vi "Patent.vi"() -> ()   [LabVIEW 2014]
uses:
  <vilib>/Instr/_visa.llb/VISA Configure Serial Port (Instr).vi
panel:
  out "flash":bool=TRUE
  out "RLCValue*":dbl=0.01
  out "Offset":string="0,00V"
  out "F4":bool
  out "F3":bool=TRUE
  out "F2":bool
  out "F1":bool
  out "Frequency":string="1kHz"
  out "Level":string="1,00V"
  out "DQValue":string="-0,0633   "
  out "RLCValue":string="0,01 pF"
  in  "Menu":bool
  in  "Down":bool
  in  ">0<":bool
  in  "F4":bool
  in  "Right":bool
  in  "Enter":bool
  in  "Left":bool
  in  "F3":bool
  in  "Z/T":bool
  in  "Up":bool
  in  "I":bool
  in  "F2":bool
  in  "R/D":bool
  in  "L/Q":bool
  in  "C/D":bool
  in  "F1":bool
  out "Ошибка связи":bool
  out "DQ":string="D"
  out "Корректный  пакет":bool=TRUE
  in  "Stop":bool
  out "Level":dbl=1.0
  out "Limit":string="A 10MOm"
  out "RLC":string="Cp"
  # "Измеритель иммитанса Е7-20"
  # "МНИПИ"
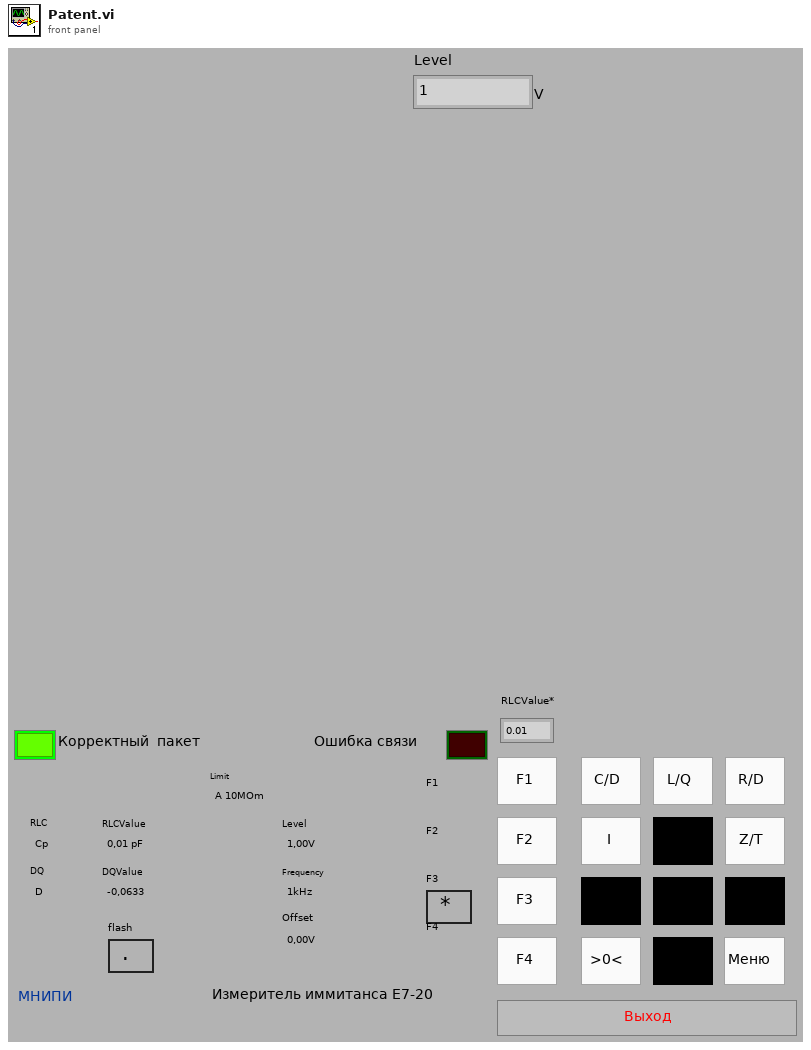
[diagram p1: front panel]
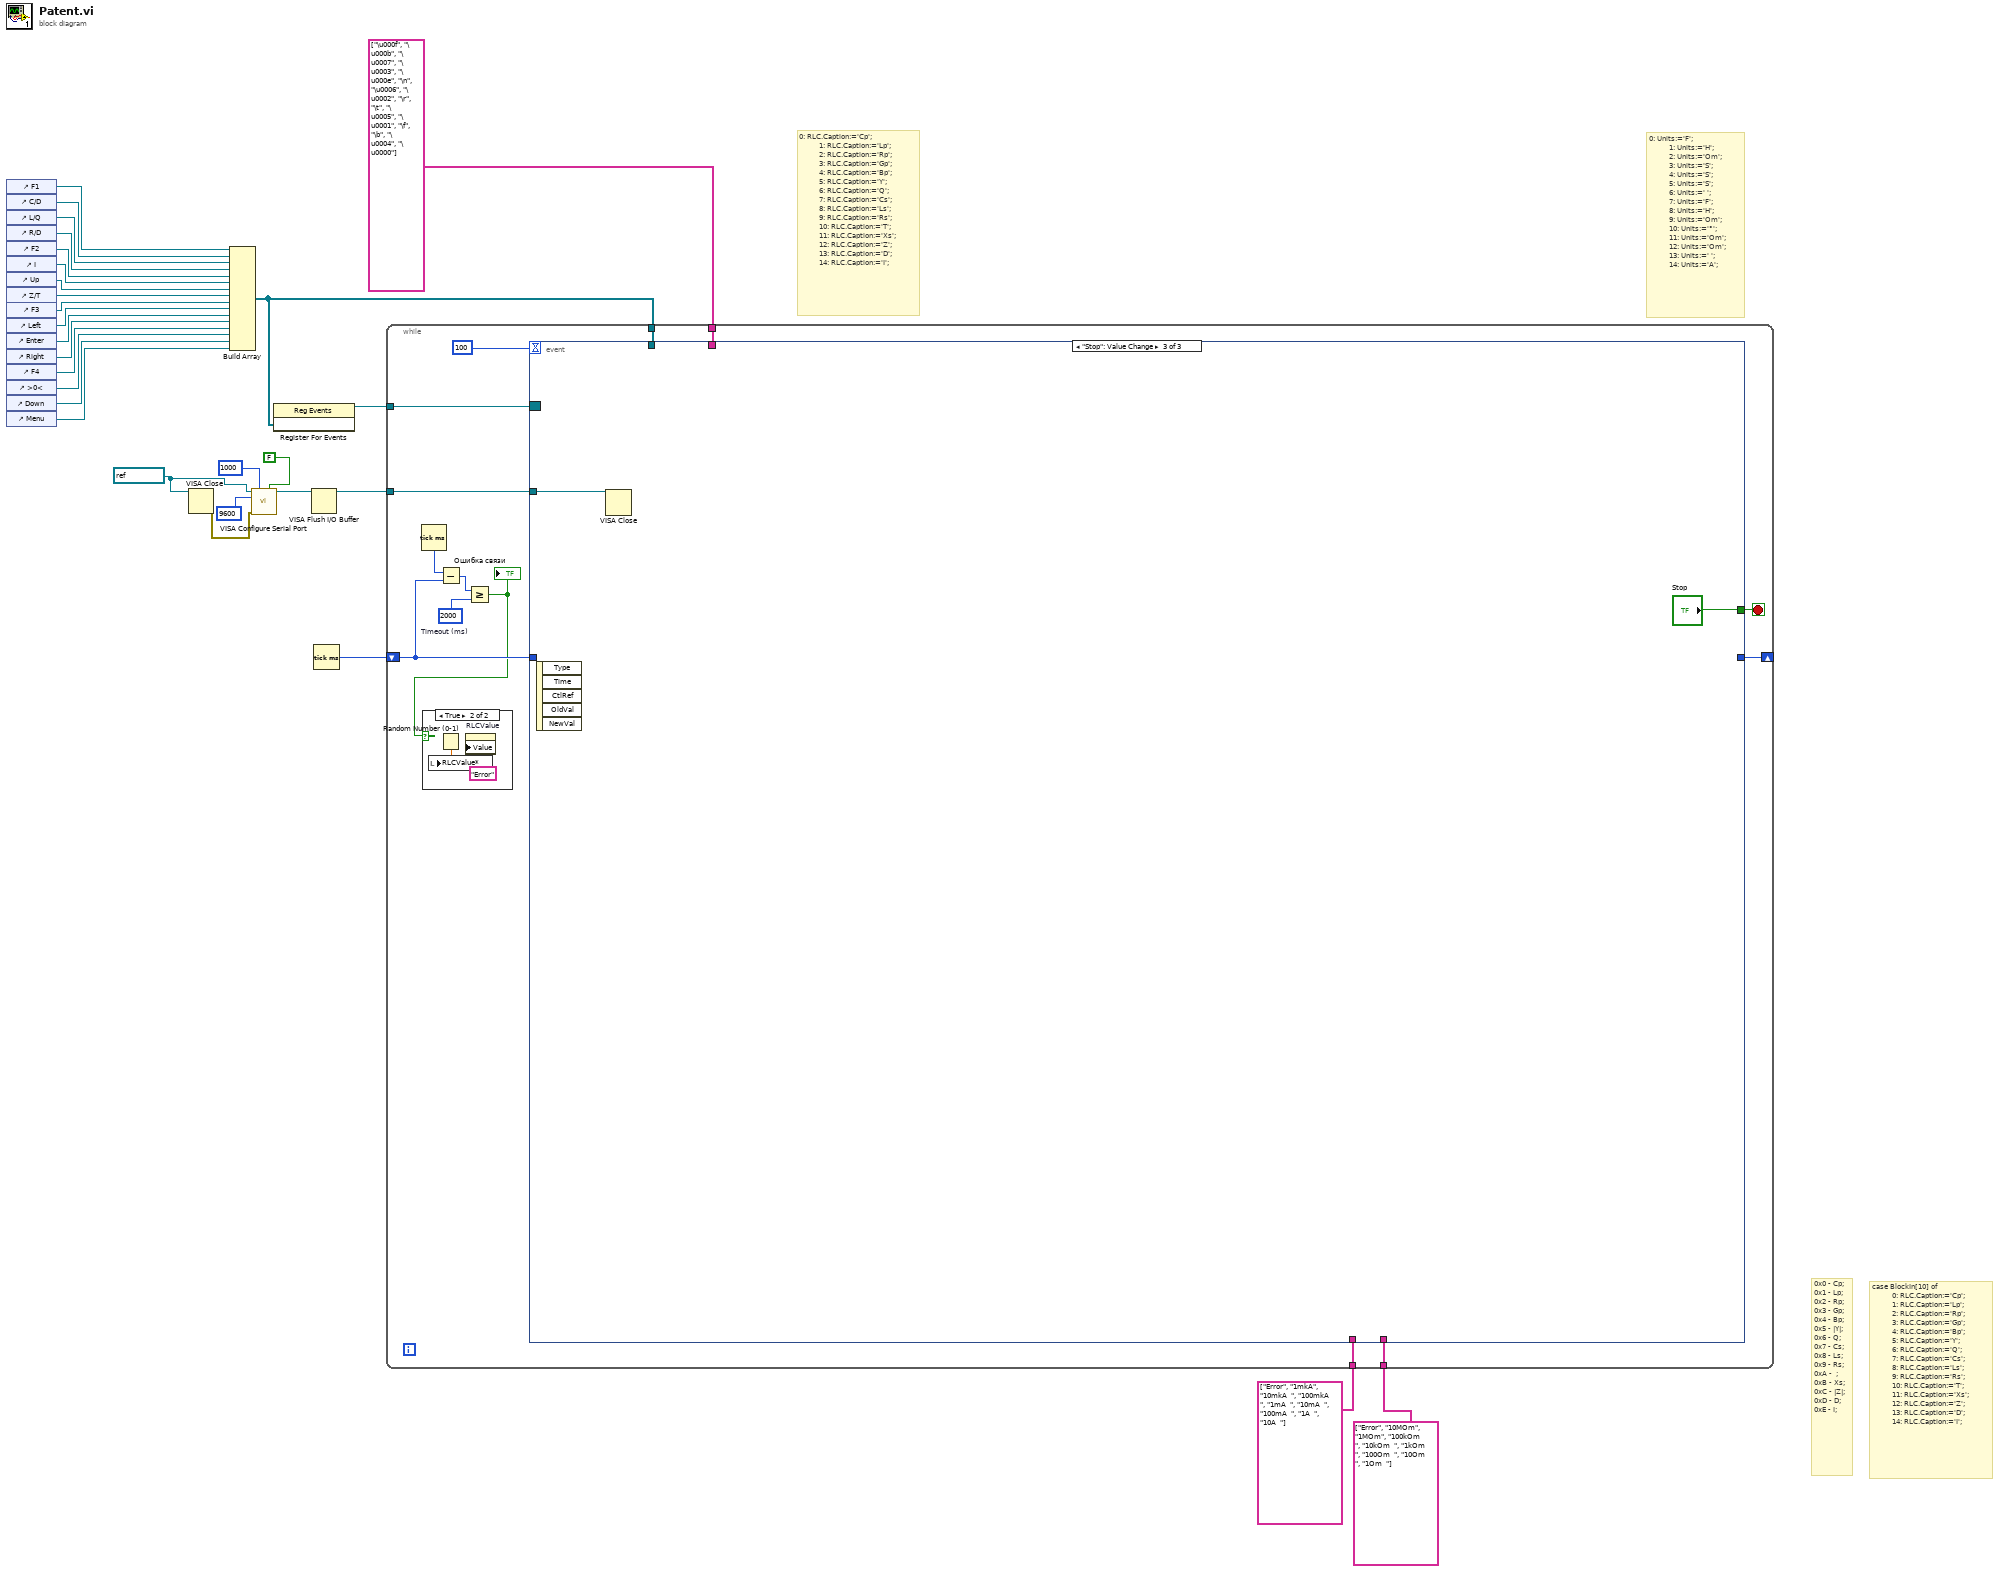
[diagram p0: block diagram]
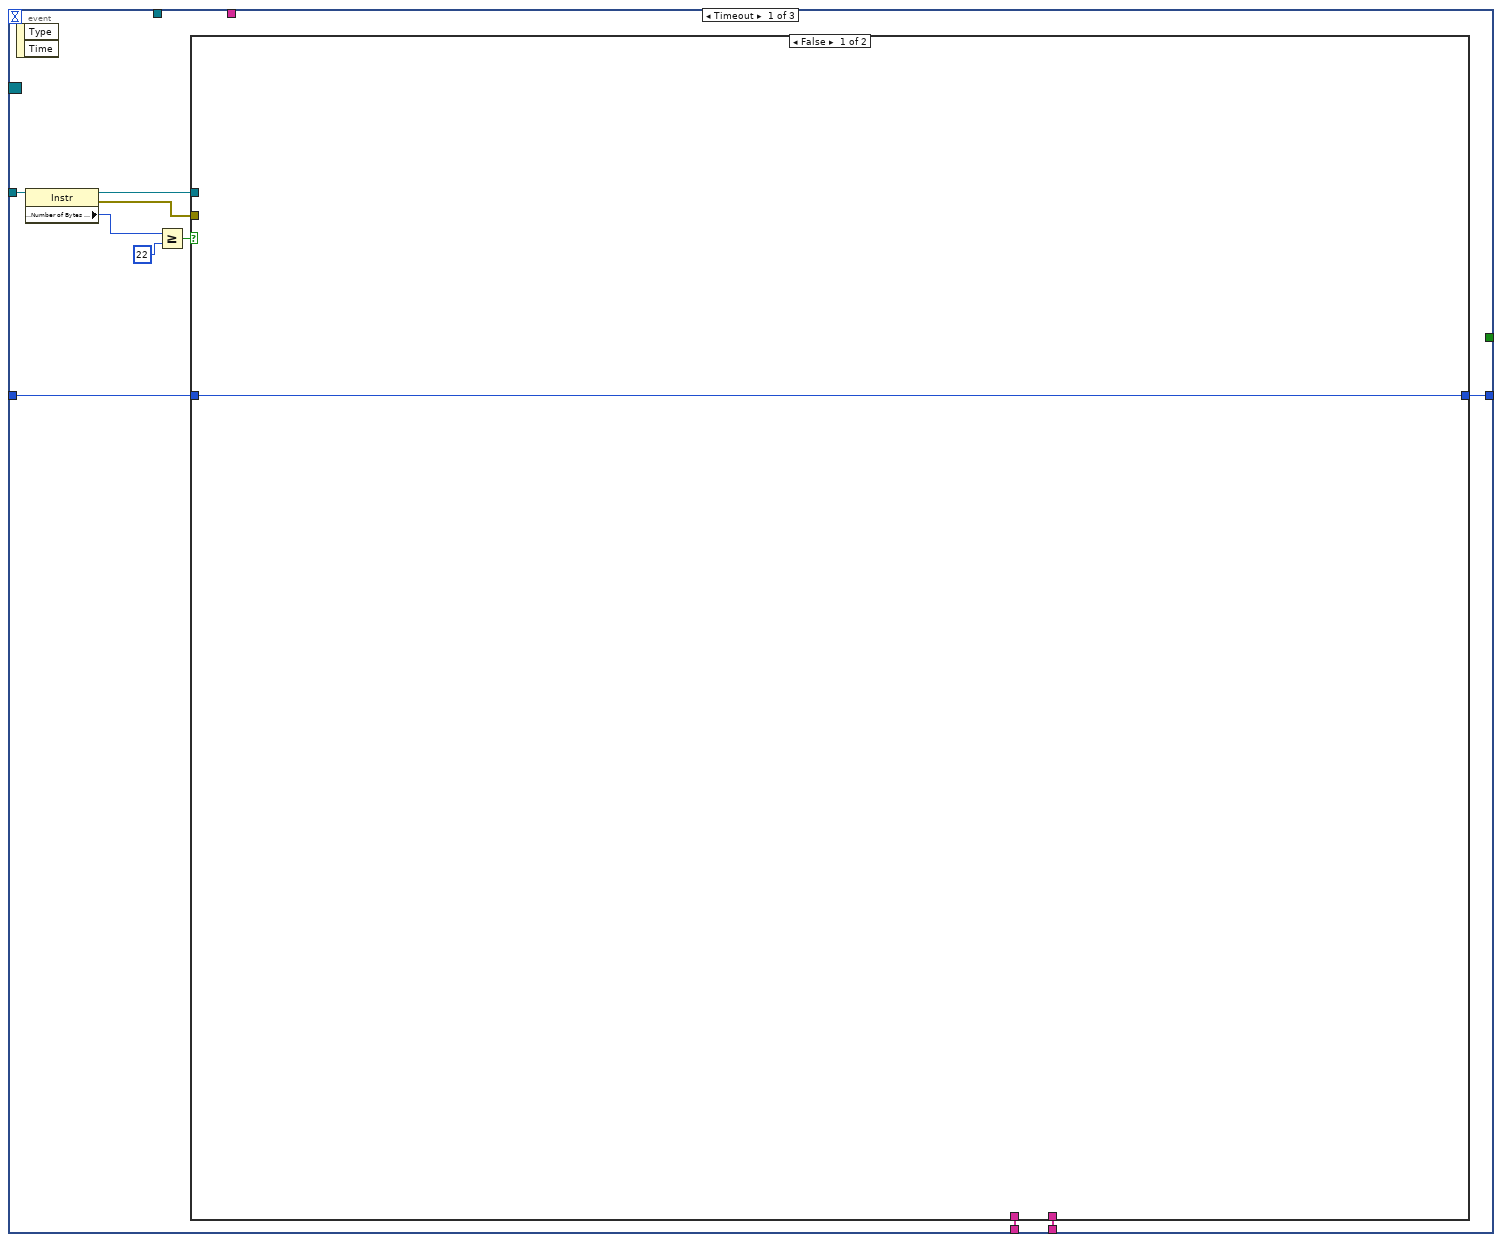
[diagram p3: hidden frame]
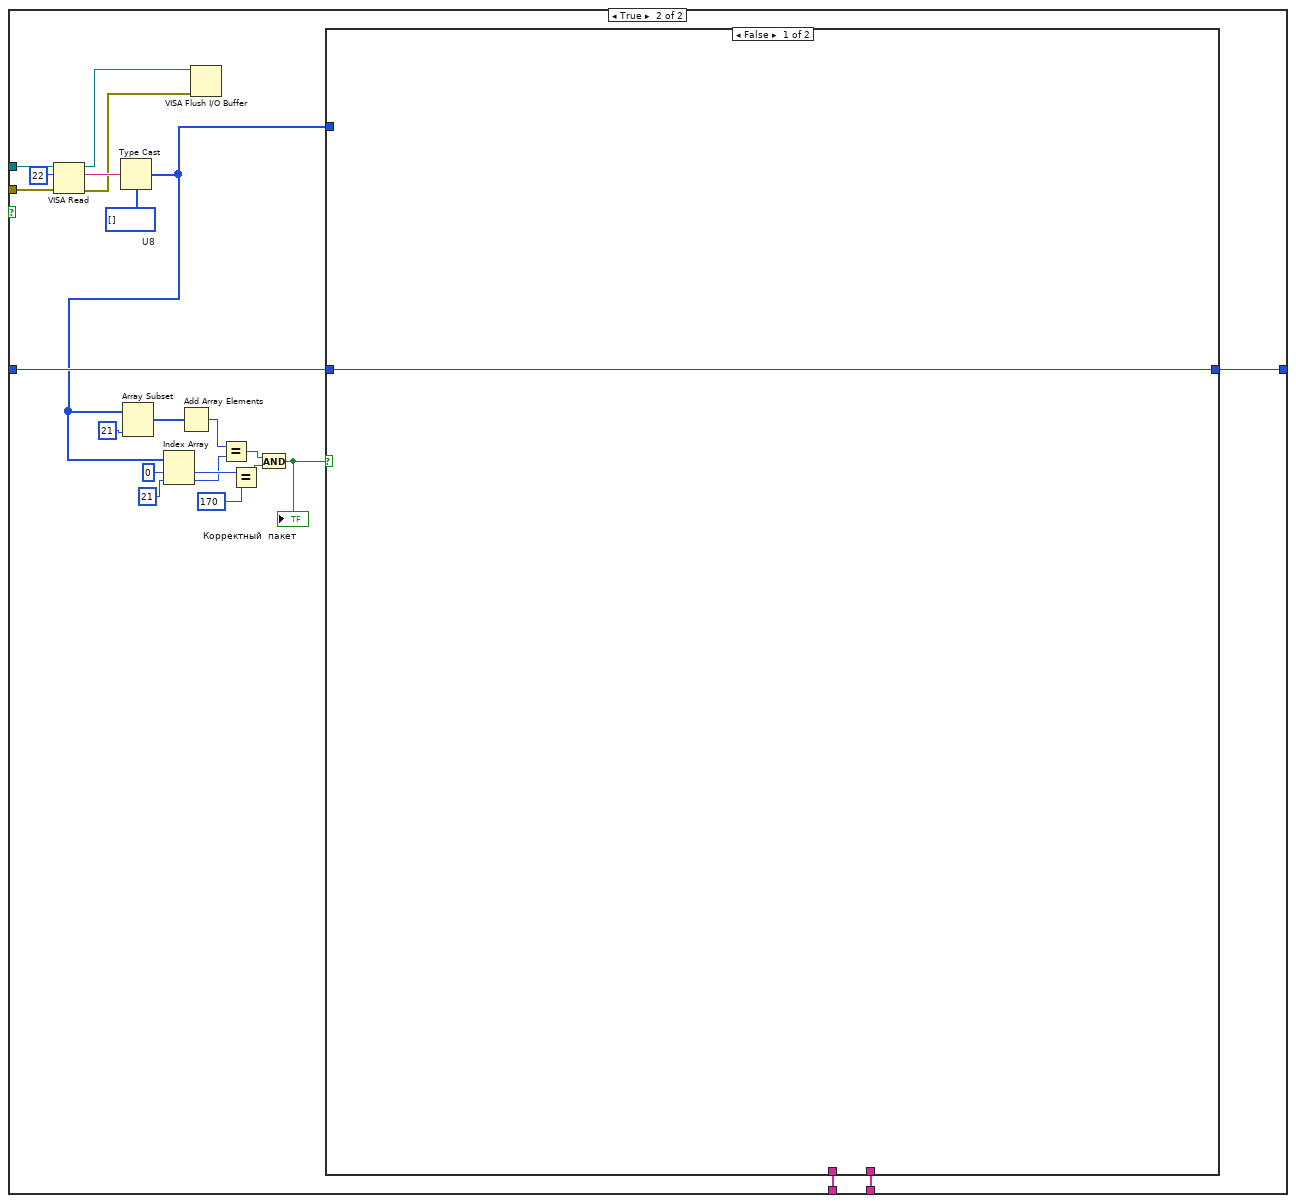
[diagram p4: hidden frame]
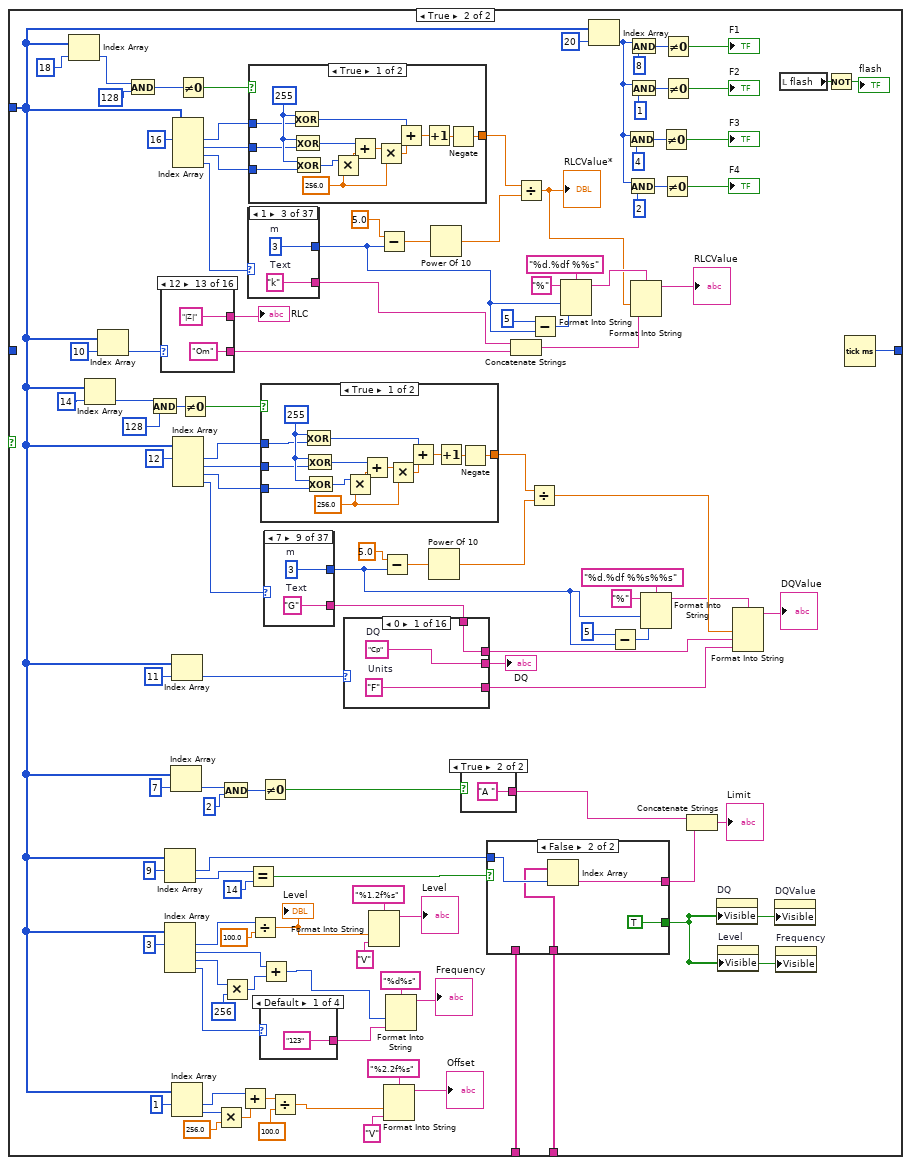
[diagram p5: hidden frame]
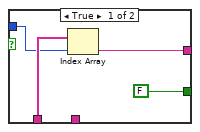
[diagram p6: hidden frame]
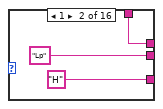
[diagram p7: hidden frame]
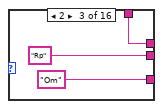
[diagram p8: hidden frame]
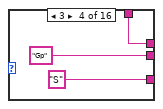
[diagram p9: hidden frame]
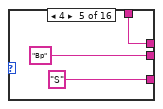
[diagram p10: hidden frame]
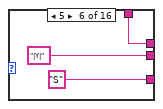
[diagram p11: hidden frame]
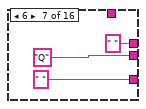
[diagram p12: hidden frame]
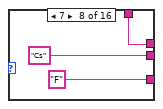
[diagram p13: hidden frame]
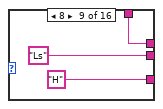
[diagram p14: hidden frame]
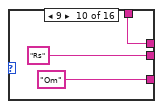
[diagram p15: hidden frame]
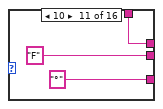
[diagram p16: hidden frame]
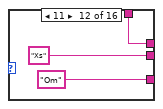
[diagram p17: hidden frame]
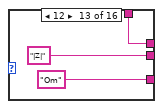
[diagram p18: hidden frame]
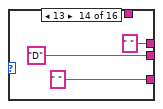
[diagram p19: hidden frame]
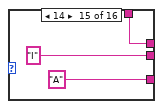
[diagram p20: hidden frame]
diagram:
  w4 = refnum<visa-resource-name> "COM1" ("VISA resource name")
  # "0: RLC.Caption:='Cp';\n          1: RLC.Caption:='Lp';\n          2: RLC.Caption:='Rp';\n          3: RLC.Caption:='Gp';\n          4: RLC.Caption:='Bp';\n          5: RLC.Caption:='Y';\n          6: RLC.Caption:='Q';\n          7: RLC.Caption:='Cs';\n          8: RLC.Caption:='Ls';\n          9: RLC.Caption:='Rs';\n          10: RLC.Caption:='T';\n          11: RLC.Caption:='Xs';\n          12: RLC.Caption:='Z';\n          13: RLC.Caption:='D';\n          14: RLC.Caption:='I';"
  # "0: Units:='F';\n          1: Units:='H';\n          2: Units:='Om';\n          3: Units:='S';\n          4: Units:='S';\n          5: Units:='S';\n          6: Units:=' ';\n          7: Units:='F';\n          8: Units:='H';\n          9: Units:='Om';\n          10: Units:='°';\n          11: Units:='Om';\n          12: Units:='Om';\n          13: Units:=' ';\n          14: Units:='A';"
  # "case BlockIn[10] of\n          0: RLC.Caption:='Cp';\n          1: RLC.Caption:='Lp';\n          2: RLC.Caption:='Rp';\n          3: RLC.Caption:='Gp';\n          4: RLC.Caption:='Bp';\n          5: RLC.Caption:='Y';\n          6: RLC.Caption:='Q';\n          7: RLC.Caption:='Cs';\n          8: RLC.Caption:='Ls';\n          9: RLC.Caption:='Rs';\n          10: RLC.Caption:='T';\n          11: RLC.Caption:='Xs';\n          12: RLC.Caption:='Z';\n          13: RLC.Caption:='D';\n          14: RLC.Caption:='I';"
  # "0х0 - Ср;\n0х1 - Lp;\n0x2 - Rp;\n0x3 - Gp;\n0x4 - Bp;\n0x5 - |Y|;\n0x6 - Q;\n0x7 - Cs;\n0x8 - Ls;\n0x9 - Rs;\n0xA -  ;\n0xB - Xs;\n0xC - |Z|;\n0xD - D;\n0xE - I;"
  n1 = control-ref of="F1"() -> (w22:refnum<vi>)
  n2 = control-ref of="C/D"() -> (w21:refnum<vi>)
  n3 = control-ref of="L/Q"() -> (w20:refnum<vi>)
  n4 = control-ref of="R/D"() -> (w19:refnum<vi>)
  n5 = control-ref of="F2"() -> (w18:refnum<vi>)
  n6 = control-ref of="I"() -> (w17:refnum<vi>)
  n7 = control-ref of="Up"() -> (w16:refnum<vi>)
  n8 = control-ref of="Z/T"() -> (w15:refnum<vi>)
  n9 = control-ref of="F3"() -> (w14:refnum<vi>)
  n10 = control-ref of="Left"() -> (w13:refnum<vi>)
  n11 = control-ref of="Enter"() -> (w12:refnum<vi>)
  n12 = control-ref of="Right"() -> (w11:refnum<vi>)
  n13 = control-ref of="F4"() -> (w10:refnum<vi>)
  n14 = control-ref of=">0<"() -> (w9:refnum<vi>)
  n15 = control-ref of="Down"() -> (w8:refnum<vi>)
  n16 = control-ref of="Menu"() -> (w7:refnum<vi>)
  n17 = VISA Close(VISA resource name=w4) -> (error out=w3:errorcluster)  [unwired: 1 in]
  n18 = Build Array(w22, w21, w20, w19, w18, w17, w16, w15, w14, w13, w12, w11, w10, w9, w8, w7) -> (w6:refnum<vi>[])
  n19 = call-poly "VISA Configure Serial Port"("VISA resource name"=w4, "timeout (10sec)"=u32 1000, "Enable Termination\nChar (T)"=FALSE ("Enable Termination\nChar (T)"), "baud rate (9600)"=u32 9600, "error in (no error)"=w3) -> ("VISA resource name out"=w2:refnum<visa-resource-name>)  [unwired: 9 in, 1 out]
  n20 = register-events(w6) -> (reference out=w23:refnum<event-registration>)  [unwired: 2 in, 1 out]
  n21 = VISA Flush I/O Buffer(VISA resource name=w2) -> (VISA resource name out=w1:refnum<visa-resource-name>)  [unwired: 2 in, 1 out]
  n22 = Tick Count (ms)() -> (millisecond timer value=w24:u32)
  n23 = while {
    tunnel: w1 -> [w42]
    tunnel: string[] ["Error", "1mkA", "10mkA  ", "100mkA  ", "1mA  ", "10mA  ", "100mA  ", "1A  ", "10A  "] -> [w41]
    tunnel: string[] ["Error", "10MOm", "1MOm", "100kOm  ", "10kOm  ", "1kOm  ", "100Om  ", "10Om  ", "1Om  "] -> [w40]
    shift-right: [w38] -> _
    shift-left: w24 -> [w34]
    tunnel: w23 -> [w33]
    tunnel: w6 -> [w32]
    tunnel: string[] ["\u000f", "\u000b", "\u0007", "\u0003", "\u000e", "\n", "\u0006", "\u0002", "\r", "\t", "\u0005", "\u0001", "\f", "\b", "\u0004", "\u0000"] -> [w31]
    stop <- w39 stop-if-true
    w37 = u32 2000  # Timeout (ms)
    n24 = Tick Count (ms)() -> (millisecond timer value=w35:u32)
    n25 = Subtract(x=w35, y=w34) -> (x-y=w36:u32)
    n26 = Greater Or Equal?(x=w36, y=w37) -> (x >= y?=w30:bool)
    "Ошибка связи" <- w30
    n27 = case shown="True" w30 {
      frame False {
      }
      frame True {
        n28 = Random Number (0-1)() -> (number: 0 to 1=w44:dbl)
        n29 = local write "RLCValue*"(w44) -> ()
        n30 = property on="RLCValue" class="Str"("Value"="Error" ("RLCValue")) -> ()  [unwired: 2 in, 2 out]
      }
    }
    n31 = event shown="[2] \"Stop\": Value Change" {
      selector: w33 -> [_ _ _]
      dyn-events: _ -> [_ _ _]
      timeout: 100 -> [_ _ _]
      tunnel: w42 -> [w51 w483 w488]
      tunnel: w41 -> [w50 _ _]
      tunnel: w40 -> [w49 _ _]
      tunnel: [_ _ "Stop"] -> w39
      tunnel: w34 -> [w47 _ _]
      tunnel: [w46 _ _] -> w38
      tunnel: w32 -> [_ w487 _]
      tunnel: w31 -> [_ w485 _]
      event Timeout {
        n32 = event-data() -> ()  [unwired: 1 in, 2 out]
        n33 = property class="Instr"(reference=w51) -> (reference out=w52:refnum<visa-resource-name>, error out=w48:errorcluster, "Serial Settings:Number of Bytes at Serial Port"=w55:u32)  [unwired: 1 in]
        n34 = Greater Or Equal?(x=w55, y=u32 22) -> (x >= y?=w53:bool)
        n35 = case shown="False" w53 {
          tunnel: w52 -> [_ w79]
          tunnel: w50 -> [_ w64]
          tunnel: w49 -> [_ w63]
          tunnel: w48 -> [_ w62]
          tunnel: w47 -> [w56 w61]
          tunnel: [w56 w60] -> w46
          frame False {
          }
          frame True {
            w76 = u8[] []  # U8
            n36 = VISA Read(VISA resource name=w79, byte count=u32 22, error in (no error)=w62) -> (VISA resource name out=w66:refnum<visa-resource-name>, read buffer=w77:string, error out=w65:errorcluster)  [unwired: 1 out]
            n37 = Type Cast(type=w76, x=w77) -> (*(type *) &x=w57:u8[])
            n38 = Array Subset(array=w57, length=21) -> (w59:u8[])  [unwired: 1 in]
            n39 = Index Array(array=w57, index #1=0 ("index"), index #2=21 ("index")) -> (element #1=w73:u8, element #2=w71:u8)
            n40 = Add Array Elements(numeric array=w59) -> (sum=w70:u8)
            n41 = VISA Flush I/O Buffer(VISA resource name=w66, error in (no error)=w65) -> ()  [unwired: 1 in, 2 out]
            n42 = Equal?(x=w70, y=w71) -> (x = y?=w68:bool)
            n43 = Equal?(x=w73, y=u8 170) -> (x = y?=w69:bool)
            n44 = And(x=w68, y=w69) -> (x .and. y?=w67:bool)
            "Корректный  пакет" <- w67
            n45 = case shown="False" w67 {
              tunnel: w57 -> [_ w103]
              tunnel: w64 -> [_ w138]
              tunnel: w63 -> [_ w137]
              tunnel: w61 -> [w80 _]
              tunnel: [w80 w123] -> w60
              frame False {
              }
              frame True {
                n46 = Index Array(array=w103, index=18) -> (element=w196:u8)
                n47 = Index Array(array=w103, index=14) -> (element=w182:u8)
                n48 = Index Array(array=w103, index=10) -> (element=w134:u8)
                n49 = And(x=w196, y=u8 128) -> (x .and. y?=w194:u8)
                n50 = And(x=w182, y=u8 128) -> (x .and. y?=w185:u8)
                n51 = case shown="12" w134 {
                  tunnel: [w254 "Lp" "Rp" "Gp" "Bp" "|Y|" "Q" "Cs" "Ls" "Rs" "F" "Xs" "|Z|" "D" "I" w283] -> w143
                  tunnel: [w253 "H" "Om" "S" "S" "S" " " "F" "H" "Om" "°" "Om" "Om" " " "A" w283] -> w84
                  frame 0 {
                    w253 = "F"  # Units
                    w254 = "Cp"  # RLC
                  }
                  frame 1 {
                  }
                  frame 2 {
                  }
                  frame 3 {
                  }
                  frame 4 {
                  }
                  frame 5 {
                  }
                  frame 6 {
                  }
                  frame 7 {
                  }
                  frame 8 {
                  }
                  frame 9 {
                  }
                  frame 10 {
                  }
                  frame 11 {
                  }
                  frame 12 {
                  }
                  frame 13 {
                  }
                  frame 14 {
                  }
                  frame Default {
                    w283 = "?"
                  }
                }
                "RLC" <- w143
                n52 = Index Array(array=w103, index #1=9 ("index")) -> (element #1=w162:u8, element #2=w164:u8)  [unwired: 1 in]
                n53 = Index Array(array=w103, index #1=3 ("index")) -> (element #1=w157:u8, element #2=w154:u8, element #3=w153:u8, element #4=w151:u8)  [unwired: 3 in]
                n54 = Index Array(array=w103, index=7) -> (element=w169:u8)
                n55 = Index Array(array=w103, index=11) -> (element=w142:u8)
                n56 = Index Array(array=w103, index #1=1 ("index")) -> (element #1=w147:u8, element #2=w146:u8)  [unwired: 1 in]
                n57 = Index Array(array=w103, index #1=16 ("index")) -> (element #1=w191:u8, element #2=w192:u8, element #3=w193:u8, element #4=w136:u8)  [unwired: 3 in]
                n58 = Index Array(array=w103, index #1=12 ("index")) -> (element #1=w179:u8, element #2=w178:u8, element #3=w177:u8, element #4=w176:u8)  [unwired: 3 in]
                n59 = Not Equal To 0?(x=w194) -> (x != 0?=w189:bool)
                n60 = Not Equal To 0?(x=w185) -> (x != 0?=w181:bool)
                n61 = Multiply(x=w146, y=256.0 ("x")) -> (x*y=w148:dbl)
                n62 = And(x=w169, y=u8 2) -> (x .and. y?=w167:u8)
                n63 = Multiply(x=w153, y=256 ("x")) -> (x*y=w155:i32)
                n64 = Add(x=w147, y=w148) -> (x+y=w145:dbl)
                n65 = case shown="1" w136 {
                  tunnel: [u8 0 ("m") w389 w391 w393 w395 w397 w399 w401 w403 w405 w407 w409 w411 w413 w415 w417 w419 w421 w423 w425 w427 w429 w431 w433 w435 w437 w439 w441 w443 w445 w447 w449 w451 w453 w455 w457 w459] -> w118
                  tunnel: ["?" ("Text") w388 w390 w392 w394 w396 w398 w400 w402 w404 w406 w408 w410 w412 w414 w416 w418 w420 w422 w424 w426 w428 w430 w432 w434 w436 w438 w440 w442 w444 w446 w448 w450 w452 w454 w456 w458] -> w85
                  frame Default {
                  }
                  frame 0 {
                    w388 = "k"  # Text
                    w389 = u8 2  # m
                  }
                  frame 1 {
                    w390 = "k"  # Text
                    w391 = u8 3  # m
                  }
                  frame 2 {
                    w392 = "k"  # Text
                    w393 = u8 4  # m
                  }
                  frame 3 {
                    w394 = "M"  # Text
                    w395 = u8 2  # m
                  }
                  frame 4 {
                    w396 = "M"  # Text
                    w397 = u8 3  # m
                  }
                  frame 5 {
                    w398 = "M"  # Text
                    w399 = u8 4  # m
                  }
                  frame 6 {
                    w400 = "G"  # Text
                    w401 = u8 2  # m
                  }
                  frame 7 {
                    w402 = "G"  # Text
                    w403 = u8 3  # m
                  }
                  frame 8 {
                    w404 = "G"  # Text
                    w405 = u8 4  # m
                  }
                  frame 9 {
                    w406 = "T"  # Text
                    w407 = u8 2  # m
                  }
                  frame 10 {
                    w408 = "T"  # Text
                    w409 = u8 3  # m
                  }
                  frame 11 {
                    w410 = "T"  # Text
                    w411 = u8 4  # m
                  }
                  frame 12 {
                    w412 = "T"  # Text
                    w413 = u8 2  # m
                  }
                  frame 13 {
                    w414 = "T"  # Text
                    w415 = u8 3  # m
                  }
                  frame 14 {
                    w416 = "T"  # Text
                    w417 = u8 4  # m
                  }
                  frame 235 {
                    w418 = "f"  # Text
                    w419 = u8 2  # m
                  }
                  frame 236 {
                    w420 = "f"  # Text
                    w421 = u8 3  # m
                  }
                  frame 237 {
                    w422 = "f"  # Text
                    w423 = u8 4  # m
                  }
                  frame 238 {
                    w424 = "f"  # Text
                    w425 = u8 2  # m
                  }
                  frame 239 {
                    w426 = "f"  # Text
                    w427 = u8 3  # m
                  }
                  frame 240 {
                    w428 = "f"  # Text
                    w429 = u8 4  # m
                  }
                  frame 241 {
                    w430 = "p"  # Text
                    w431 = u8 2  # m
                  }
                  frame 242 {
                    w432 = "p"  # Text
                    w433 = u8 3  # m
                  }
                  frame 243 {
                    w434 = "p"  # Text
                    w435 = u8 4  # m
                  }
                  frame 244 {
                    w436 = "n"  # Text
                    w437 = u8 2  # m
                  }
                  frame 245 {
                    w438 = "n"  # Text
                    w439 = u8 3  # m
                  }
                  frame 246 {
                    w440 = "n"  # Text
                    w441 = u8 4  # m
                  }
                  frame 247 {
                    w442 = "mk"  # Text
                    w443 = u8 2  # m
                  }
                  frame 248 {
                    w444 = "mk"  # Text
                    w445 = u8 3  # m
                  }
                  frame 249 {
                    w446 = "mk"  # Text
                    w447 = u8 4  # m
                  }
                  frame 250 {
                    w448 = "m"  # Text
                    w449 = u8 2  # m
                  }
                  frame 251 {
                    w450 = "m"  # Text
                    w451 = u8 3  # m
                  }
                  frame 252 {
                    w452 = "m"  # Text
                    w453 = u8 4  # m
                  }
                  frame 253 {
                    w454 = " "  # Text
                    w455 = u8 2  # m
                  }
                  frame 254 {
                    w456 = " "  # Text
                    w457 = u8 3  # m
                  }
                  frame 255 {
                    w458 = " "  # Text
                    w459 = u8 4  # m
                  }
                }
                n66 = Equal?(x=w164, y=u8 14) -> (x = y?=w139:bool)
                n67 = case shown="True" w189 {
                  tunnel: w193 -> [w472 w477]
                  tunnel: w192 -> [w471 w476]
                  tunnel: w191 -> [w470 w475]
                  tunnel: [w460 w474] -> w186
                  frame True {
                    w466 = 256.0 ("x")
                    w473 = u8 255 ("x")
                    n68 = Exclusive Or(1:w470, 2:w473) -> (0:w463:u8)
                    n69 = Exclusive Or(1:w471, 2:w473) -> (0:w464:u8)
                    n70 = Exclusive Or(1:w472, 2:w473) -> (0:w465:u8)
                    n71 = Multiply(x=w465, y=w466) -> (x*y=w468:dbl)
                    n72 = Add(x=w464, y=w468) -> (x+y=w467:dbl)
                    n73 = Multiply(x=w467, y=w466) -> (x*y=w469:dbl)
                    n74 = Add(x=w463, y=w469) -> (x+y=w462:dbl)
                    n75 = Increment(x=w462) -> (x+1=w461:dbl)
                    n76 = Negate(x=w461) -> (-x=w460:dbl)
                  }
                  frame False {
                    w478 = 256.0 ("x")
                    n77 = Multiply(x=w477, y=w478) -> (x*y=w480:dbl)
                    n78 = Add(x=w476, y=w480) -> (x+y=w479:dbl)
                    n79 = Multiply(x=w479, y=w478) -> (x*y=w481:dbl)
                    n80 = Add(x=w475, y=w481) -> (x+y=w474:dbl)
                  }
                }
                n81 = Divide(x=w157, y=100.0) -> (x/y=w101:dbl)
                "Level" <- w101
                n82 = Not Equal To 0?(x=w167) -> (x != 0?=w166:bool)
                n83 = case shown="Default" w151 {
                  tunnel: ["123" ("Text") "Hz" ("Text") w286 w287] -> w97
                  frame Default {
                  }
                  frame 0 {
                  }
                  frame 3 {
                    w286 = "kHz"  # Text
                  }
                  frame 6 {
                    w287 = "MHz"  # Text
                  }
                }
                n84 = case shown="True" w181 {
                  tunnel: w177 -> [w376 w381]
                  tunnel: w178 -> [w375 w380]
                  tunnel: w179 -> [w374 w379]
                  tunnel: [w364 w378] -> w172
                  frame True {
                    w370 = 256.0 ("x")
                    w377 = u8 255 ("x")
                    n85 = Exclusive Or(1:w374, 2:w377) -> (0:w367:u8)
                    n86 = Exclusive Or(1:w375, 2:w377) -> (0:w368:u8)
                    n87 = Exclusive Or(1:w376, 2:w377) -> (0:w369:u8)
                    n88 = Multiply(x=w369, y=w370) -> (x*y=w372:dbl)
                    n89 = Add(x=w368, y=w372) -> (x+y=w371:dbl)
                    n90 = Multiply(x=w371, y=w370) -> (x*y=w373:dbl)
                    n91 = Add(x=w367, y=w373) -> (x+y=w366:dbl)
                    n92 = Increment(x=w366) -> (x+1=w365:dbl)
                    n93 = Negate(x=w365) -> (-x=w364:dbl)
                  }
                  frame False {
                    w382 = 256.0 ("x")
                    n94 = Multiply(x=w381, y=w382) -> (x*y=w384:dbl)
                    n95 = Add(x=w380, y=w384) -> (x+y=w383:dbl)
                    n96 = Multiply(x=w383, y=w382) -> (x*y=w385:dbl)
                    n97 = Add(x=w379, y=w385) -> (x+y=w378:dbl)
                  }
                }
                n98 = Add(x=w154, y=w155) -> (x+y=w96:i32)
                n99 = case shown="7" w176 {
                  tunnel: [u8 0 ("m") w293 w295 w297 w299 w301 w303 w305 w307 w309 w311 w313 w315 w317 w319 w321 w323 w325 w327 w329 w331 w333 w335 w337 w339 w341 w343 w345 w347 w349 w351 w353 w355 w357 w359 w361 w363] -> w108
                  tunnel: ["?" ("Text") w292 w294 w296 w298 w300 w302 w304 w306 w308 w310 w312 w314 w316 w318 w320 w322 w324 w326 w328 w330 w332 w334 w336 w338 w340 w342 w344 w346 w348 w350 w352 w354 w356 w358 w360 w362] -> w140
                  frame Default {
                  }
                  frame 0 {
                    w292 = "k"  # Text
                    w293 = u8 1  # m
                  }
                  frame 1 {
                    w294 = "k"  # Text
                    w295 = u8 2  # m
                  }
                  frame 2 {
                    w296 = "k"  # Text
                    w297 = u8 3  # m
                  }
                  frame 3 {
                    w298 = "M"  # Text
                    w299 = u8 4  # m
                  }
                  frame 4 {
                    w300 = "M"  # Text
                    w301 = u8 3  # m
                  }
                  frame 5 {
                    w302 = "M"  # Text
                    w303 = u8 4  # m
                  }
                  frame 6 {
                    w304 = "G"  # Text
                    w305 = u8 2  # m
                  }
                  frame 7 {
                    w306 = "G"  # Text
                    w307 = u8 3  # m
                  }
                  frame 8 {
                    w308 = "G"  # Text
                    w309 = u8 4  # m
                  }
                  frame 9 {
                    w310 = "T"  # Text
                    w311 = u8 2  # m
                  }
                  frame 10 {
                    w312 = "T"  # Text
                    w313 = u8 3  # m
                  }
                  frame 11 {
                    w314 = "T"  # Text
                    w315 = u8 4  # m
                  }
                  frame 12 {
                    w316 = "T"  # Text
                    w317 = u8 2  # m
                  }
                  frame 13 {
                    w318 = "T"  # Text
                    w319 = u8 3  # m
                  }
                  frame 14 {
                    w320 = "T"  # Text
                    w321 = u8 4  # m
                  }
                  frame 235 {
                    w322 = "f"  # Text
                    w323 = u8 2  # m
                  }
                  frame 236 {
                    w324 = "f"  # Text
                    w325 = u8 3  # m
                  }
                  frame 237 {
                    w326 = "f"  # Text
                    w327 = u8 4  # m
                  }
                  frame 238 {
                    w328 = "f"  # Text
                    w329 = u8 2  # m
                  }
                  frame 239 {
                    w330 = "f"  # Text
                    w331 = u8 3  # m
                  }
                  frame 240 {
                    w332 = "f"  # Text
                    w333 = u8 4  # m
                  }
                  frame 241 {
                    w334 = "p"  # Text
                    w335 = u8 2  # m
                  }
                  frame 242 {
                    w336 = "p"  # Text
                    w337 = u8 3  # m
                  }
                  frame 243 {
                    w338 = "p"  # Text
                    w339 = u8 4  # m
                  }
                  frame 244 {
                    w340 = "n"  # Text
                    w341 = u8 2  # m
                  }
                  frame 245 {
                    w342 = "n"  # Text
                    w343 = u8 3  # m
                  }
                  frame 246 {
                    w344 = "n"  # Text
                    w345 = u8 4  # m
                  }
                  frame 247 {
                    w346 = "mk"  # Text
                    w347 = u8 2  # m
                  }
                  frame 248 {
                    w348 = "mk"  # Text
                    w349 = u8 1  # m
                  }
                  frame 249 {
                    w350 = "mk"  # Text
                    w351 = u8 2  # m
                  }
                  frame 250 {
                    w352 = "m"  # Text
                    w353 = u8 3  # m
                  }
                  frame 251 {
                    w354 = "m"  # Text
                    w355 = u8 4  # m
                  }
                  frame 252 {
                    w356 = "m"  # Text
                    w357 = u8 1  # m
                  }
                  frame 253 {
                    w358 = " "  # Text
                    w359 = u8 2  # m
                  }
                  frame 254 {
                    w360 = " "  # Text
                    w361 = u8 3  # m
                  }
                  frame 255 {
                    w362 = " "  # Text
                    w363 = u8 4  # m
                  }
                }
                n100 = Divide(x=w145, y=100.0) -> (x/y=w92:dbl)
                n101 = case shown="0" w142 {
                  tunnel: [w208 "Lp" "Rp" "Gp" "Bp" "|Y|" "Q" "Cs" "Ls" "Rs" "F" "Xs" "|Z|" "D" "I" w252] -> w141
                  tunnel: [w207 "H" "Om" "S" "S" "S" " " "F" "H" "Om" "°" "Om" "Om" " " "A" w252] -> w105
                  tunnel: w140 -> [w206 w209 w212 w215 w218 w221 _ w227 w230 w233 w236 w239 w242 _ w248 w251]
                  tunnel: [w206 w209 w212 w215 w218 w221 " " ("Text") w227 w230 w233 w236 w239 w242 " " ("Text") w248 w251] -> w106
                  frame 0 {
                    w207 = "F"  # Units
                    w208 = "Cp"  # DQ
                  }
                  frame 1 {
                  }
                  frame 2 {
                  }
                  frame 3 {
                  }
                  frame 4 {
                  }
                  frame 5 {
                  }
                  frame 6 {
                  }
                  frame 7 {
                  }
                  frame 8 {
                  }
                  frame 9 {
                  }
                  frame 10 {
                  }
                  frame 11 {
                  }
                  frame 12 {
                  }
                  frame 13 {
                  }
                  frame 14 {
                  }
                  frame Default {
                    w252 = "?"
                  }
                }
                "DQ" <- w141
                n102 = Format Into String(format string="%1.2f%s", w101, "V" ("input 2")) -> (resulting string=→"Level":string)  [unwired: 2 in, 1 out]
                n103 = Subtract(x=5.0, y=w118) -> (x-y=w187:dbl)
                n104 = Subtract(x=5.0, y=w108) -> (x-y=w174:dbl)
                n105 = Format Into String(format string="%2.2f%s", w92, "V" ("input 2")) -> (resulting string=→"Offset":string)  [unwired: 2 in, 1 out]
                n106 = Format Into String(format string="%d%s", w96, w97) -> (resulting string=→"Frequency":string)  [unwired: 2 in, 1 out]
                n107 = Power Of 10(x=w174) -> (10^x=w171:dbl)
                n108 = Power Of 10(x=w187) -> (10^x=w122:dbl)
                n109 = case shown="True" w166 {
                  tunnel: ["   " ("Limit.Caption") "A " ("Limit.Caption")] -> w161
                  frame False {
                  }
                  frame True {
                  }
                }
                n110 = case shown="False" w139 {
                  tunnel: w162 -> [w199 w204]
                  tunnel: [w201 w205] -> w160
                  tunnel: w138 -> [w200 _]
                  tunnel: w137 -> [_ w203]
                  tunnel: [FALSE TRUE] -> w91
                  frame True {
                    n111 = Index Array(array=w200, index=w199) -> (element=w201:string)
                  }
                  frame False {
                    n112 = Index Array(array=w203, index=w204) -> (element=w205:string)
                  }
                }
                n113 = Concatenate Strings(w85, w84) -> (w83:string)
                n114 = Divide(x=w186, y=w122) -> (x/y=w113:dbl)
                "RLCValue*" <- w113
                n115 = Divide(x=w172, y=w171) -> (x/y=w114:dbl)
                n116 = Subtract(x=u8 5 ("input 2"), y=w118) -> (x-y=w119:u8)
                n117 = Format Into String(format string="%d.%df %%s", initial string="%", w118, w119) -> (resulting string=w117:string)  [unwired: 1 in, 1 out]
                n118 = Index Array(array=w103, index=20) -> (element=w124:u8)
                n119 = Subtract(x=u8 5 ("input 2"), y=w108) -> (x-y=w110:u8)
                n120 = And(x=w124, y=u8 4) -> (x .and. y?=w127:u8)
                n121 = And(x=w124, y=u8 2) -> (x .and. y?=w125:u8)
                n122 = And(x=w124, y=u8 8) -> (x .and. y?=w131:u8)
                n123 = And(x=w124, y=u8 1) -> (x .and. y?=w130:u8)
                n124 = Format Into String(format string=w117, w113, w83) -> (resulting string=→"RLCValue":string)  [unwired: 2 in, 1 out]
                n125 = Format Into String(format string="%d.%df %%s%%s", initial string="%", w108, w110) -> (resulting string=w107:string)  [unwired: 1 in, 1 out]
                n126 = Not Equal To 0?(x=w127) -> (x != 0?=→"F3":bool)
                n127 = Not Equal To 0?(x=w125) -> (x != 0?=→"F4":bool)
                n128 = Not Equal To 0?(x=w131) -> (x != 0?=→"F1":bool)
                n129 = Not Equal To 0?(x=w130) -> (x != 0?=→"F2":bool)
                n130 = Concatenate Strings(w161, w160) -> (→"Limit":string)
                n131 = property on="DQ" class="Str"("Visible"=w91) -> ()  [unwired: 2 in, 2 out]
                n132 = property on="Level" class="Str"("Visible"=w91) -> ()  [unwired: 2 in, 2 out]
                n133 = Format Into String(format string=w107, w114, w106, w105) -> (resulting string=→"DQValue":string)  [unwired: 2 in, 1 out]
                n134 = property on="DQValue" class="Str"("Visible"=w91) -> ()  [unwired: 2 in, 2 out]
                n135 = property on="Frequency" class="Str"("Visible"=w91) -> ()  [unwired: 2 in, 2 out]
                n136 = local read "flash"() -> (w81:bool)
                n137 = Not(x=w81) -> (.not. x?=→"flash":bool)
                n138 = Tick Count (ms)() -> (millisecond timer value=w123:u32)
              }
            }
          }
        }
      }
      event Value Change {
        n139 = event-data() -> ("CtlRef"=w486:refnum<vi>)  [unwired: 1 in]
        n140 = Search 1D Array(1D array=w487, element=w486) -> (index of element=w484:i32)  [unwired: 1 in]
        n141 = Index Array(array=w485, index=w484) -> (element=w482:string)
        n142 = VISA Write(VISA resource name=w483, write buffer=w482) -> ()  [unwired: 1 in, 3 out]
      }
      event "Stop": Value Change {
        n143 = event-data() -> ()  [unwired: 1 in, 5 out]
        n144 = VISA Close(VISA resource name=w488) -> ()  [unwired: 1 in, 1 out]
      }
    }
  }
